vi "Parse Keep-Alive Data.vi"(11 "Keep-Alive Data":string) -> (3 "All Scripts":T1[](array[typedef]))   [LabVIEW 2013, in "TS.lvlib"]
doc: "The keep-alive message from Python has data that looks like this:\n{'12756': False, '2112': False}\nThis VI parses the data into the data structure output."
uses:
  TS.lvlib
  LabVIEW Example/Supporting Code/Script Running.ctl
panel:
  out "substring":string
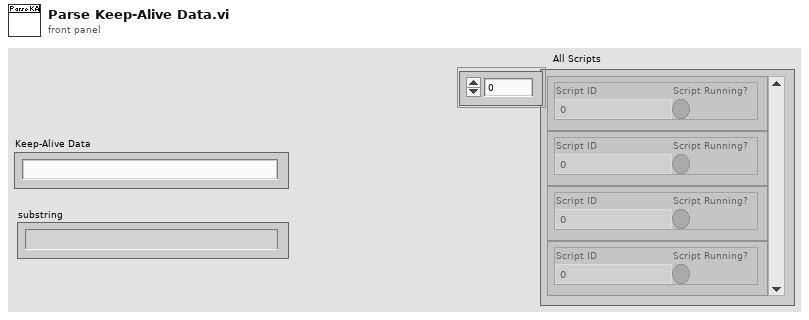
[diagram p1: front panel]
types:
  T1 = typedef "TS.lvlib/Script Running.ctl" = cluster{"Script ID":i64, "Script Running?":bool}
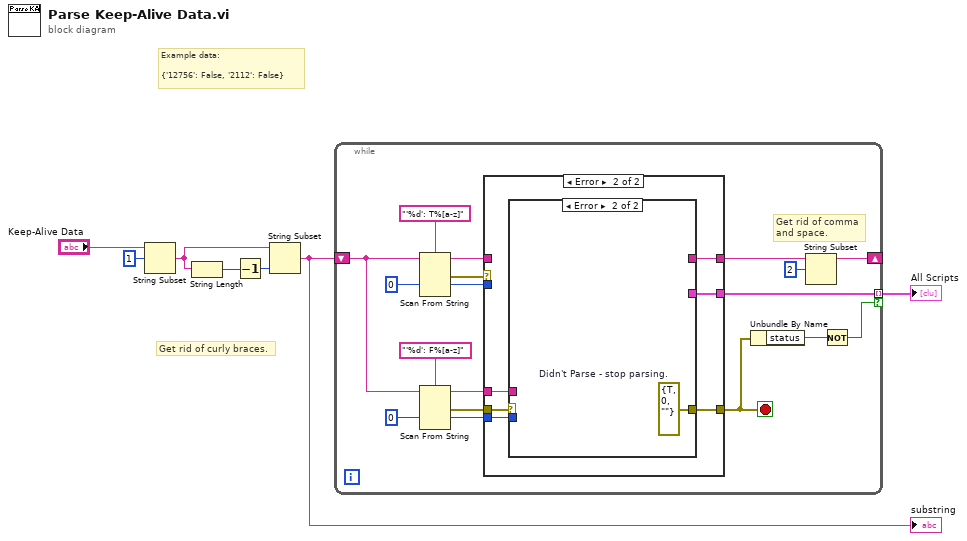
[diagram p0: block diagram]
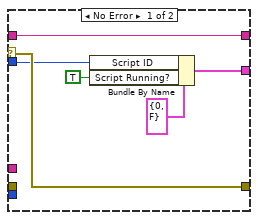
[diagram p2: hidden frame]
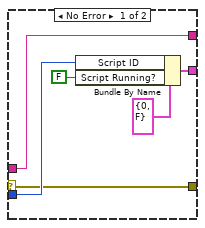
[diagram p3: hidden frame]
diagram:
  # "Get rid of curly braces."
  # "Example data:\n\n{'12756': False, '2112': False}"
  n1 = String Subset(string="Keep-Alive Data", offset (0)=1) -> (substring=w5:string)  [unwired: 1 in]
  n2 = String Length(string=w5) -> (length=w4:i32)
  n3 = Decrement(x=w4) -> (x-1=w3:i32)
  n4 = String Subset(string=w5, length (rest)=w3) -> (substring=w2:string)  [unwired: 1 in]
  "substring" <- w2
  n5 = while {
    shift-right: [w9] -> _
    shift-left: w2 -> [w23]
    tunnel: [w13] -> w1 mode=indexing if=w10
    stop <- w12 stop-if-true
    # "Get rid of comma\nand space."
    n6 = Scan From String(format string="'%d': T%[a-z]" ("regular expression"), input string=w23, default 1=i64 0) -> (remaining string=w22:string, error out=w20:errorcluster, output 1=w18:i64)  [unwired: 4 in, 1 out]
    n7 = Scan From String(format string="'%d': F%[a-z]" ("regular expression"), input string=w23, default 1=i64 0) -> (remaining string=w21:string, error out=w15:errorcluster, output 1=w16:i64)  [unwired: 4 in, 1 out]
    n8 = case shown="Error" w20 {
      selector: w20 -> [w31 _]
      tunnel: w22 -> [w30 _]
      tunnel: w21 -> [_ w36]
      tunnel: w18 -> [w28 _]
      tunnel: w16 -> [_ w35]
      tunnel: w15 -> [_ w37]
      tunnel: [w31 w32] -> w12
      tunnel: [w30 w33] -> w14
      tunnel: [w26 w34] -> w13
      frame No Error {
        n9 = Bundle By Name(cluster=T1 {"Script ID"=0, "Script Running?"=FALSE} ("Script Running?"), "Script ID"=w28, "Script Running?"=TRUE) -> (w26:T1)
      }
      frame Error {
        n10 = case shown="Error" w37 {
          selector: w37 -> [w38 _]
          tunnel: w36 -> [w39 _]
          tunnel: w35 -> [w41 _]
          tunnel: [w40 _] -> w34
          tunnel: [w39 _] -> w33
          tunnel: [w38 w44] -> w32
          frame No Error {
            n11 = Bundle By Name(cluster=T1 {"Script ID"=0, "Script Running?"=FALSE} ("Script Running?"), "Script ID"=w41, "Script Running?"=FALSE) -> (w40:T1)
          }
          frame Error {
            w44 = errorcluster {"status"=TRUE, "code"=0, "source"=""}  # Didn't Parse - stop parsing.
          }
        }
      }
    }
    n12 = Unbundle By Name(w12) -> ("status"=w11:bool)
    n13 = String Subset(string=w14, offset (0)=2) -> (substring=w9:string)  [unwired: 1 in]
    n14 = Not(x=w11) -> (.not. x?=w10:bool)
  }
  "All Scripts" <- w1
